vi "welcome.vi"   [LabVIEW 2018]
uses:
  user32.dll
types:
  T1 = enum32{"Invalid", "Standard", "Closed", "Hidden", "Minimized", "Maximized"}
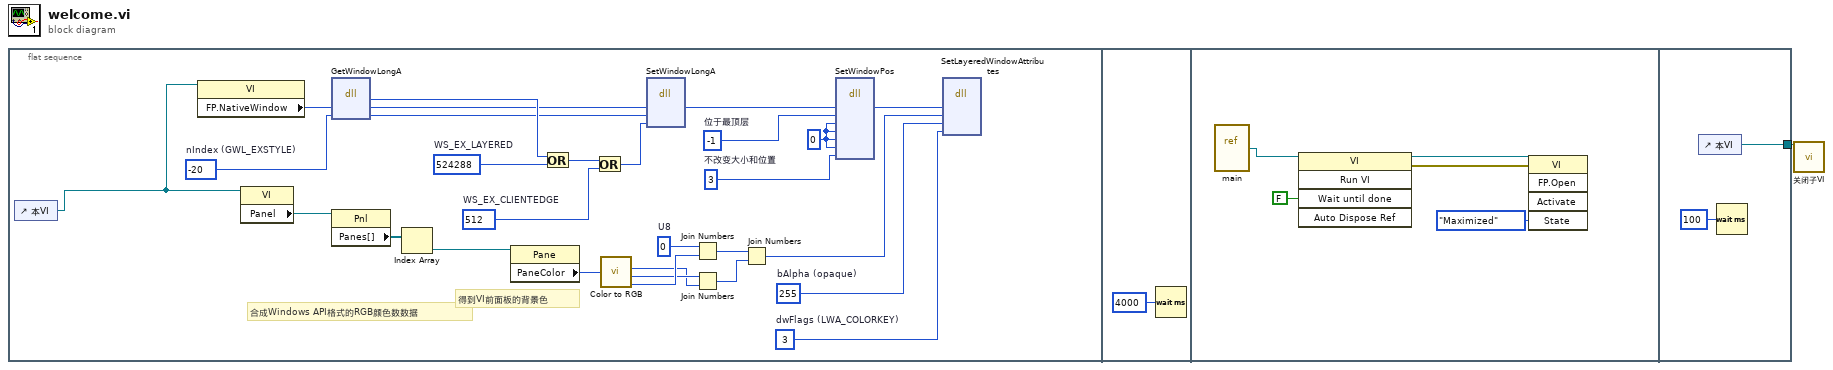
[diagram p0: block diagram]
diagram:
  n1 = flat-sequence {
    tunnel: [w36] -> w1
    frame #0 {
      w26 = 512  # WS_EX_CLIENTEDGE
      w22 = 3  # 不改变大小和位置
      w25 = 0 ("nIndex")
      w21 = -1  # 位于最顶层
      w3 = 255  # bAlpha (opaque)
      w2 = 3  # dwFlags (LWA_COLORKEY)
      w10 = u8 0  # U8
      w18 = 524288  # WS_EX_LAYERED
      w19 = -20  # nIndex (GWL_EXSTYLE)
      # "合成Windows API格式的RGB颜色数数据"
      # "得到VI前面板的背景色"
      n2 = control-ref of="本VI"() -> (w29:refnum<vi>)
      n3 = property class="VI"(reference=w29) -> ("FP.NativeWindow"=w20:u64)  [unwired: 1 in, 2 out]
      n4 = property class="VI"(reference=w29) -> ("Panel"=w5:refnum<vi>)  [unwired: 1 in, 2 out]
      n5 = dll-call lib="user32.dll" fn="GetWindowLongA"("handle"=w20, "nIndex"=w19) -> ("返回类型"=w17:i32, "handle"=w16:i32, "nIndex"=w15:i32)  [unwired: 3 in, 2 out]
      n6 = property class="Pnl"(reference=w5) -> ("Panes[]"=w6:refnum<vi>[])  [unwired: 1 in, 2 out]
      n7 = Index Array(array=w6) -> (element=w7:refnum<vi>)  [unwired: 1 in]
      n8 = property class="Pane"(reference=w7) -> ("PaneColor"=w11:u32)  [unwired: 1 in, 2 out]
      n9 = Or(x=w17, y=w18) -> (x .or. y?=w27:i32)
      n10 = Or(x=w27, y=w26) -> (x .or. y?=w28:i32)
      n11 = call <vilib>:"Color to RGB.vi"("Color"=w11) -> ("R"=w12:u8, "G"=w13:u8, "B"=w14:u8)  [unwired: 1 out]
      n12 = dll-call lib="USER32.DLL" fn="SetWindowLongA" label="SetWindowLong"("handle"=w16, "nIndex"=w15, "dwNewLong"=w28) -> ("handle"=w23:i32)  [unwired: 5 in, 3 out]
      n13 = Join Numbers(hi=w10, lo=w14) -> ((hi.lo)=w9:u16)
      n14 = Join Numbers(hi=w13, lo=w12) -> ((hi.lo)=w8:u16)
      n15 = Join Numbers(hi=w9, lo=w8) -> ((hi.lo)=w4:u32)
      n16 = dll-call lib="USER32.DLL" fn="SetWindowPos"("hWnd"=w23, "hWndInsertAfter"=w21, "x"=w25, "y"=w25, "cx"=w25, "cy"=w25, "wFlags"=w22) -> ("hWnd"=w24:i32)  [unwired: 9 in, 3 out]
      n17 = dll-call lib="USER32.DLL" fn="SetLayeredWindowAttributes" label="SetLayerdWindowAttributs"("handle"=w24, "crkey"=w4, "bAlpha"=w3, "dwFlags"=w2) -> ()  [unwired: 7 in, 3 out]
    }
    frame #1 {
      n18 = Wait (ms)(milliseconds to wait=u32 4000 ("等待时间（毫秒）")) -> ()  [unwired: 1 out]
    }
    frame #2 {
      n19 = vi-ref "main.vi"() -> (w31:refnum<vi>)
      n20 = invoke class="VI" method="Run VI"(reference=w31, "Wait until done"=FALSE ("结束前等待")) -> (reference out=w34:refnum<vi>, error out=w35:errorcluster)  [unwired: 3 in, 3 out]
      n21 = invoke class="VI" method="FP.Open"(reference=w34, error in=w35, "State"=T1."Maximized" ("状态")) -> ()  [unwired: 2 in, 5 out]
    }
    frame #3 {
      n22 = control-ref of="本VI"() -> (w36:refnum<vi>)
      n23 = Wait (ms)(milliseconds to wait=u32 100 ("等待时间（毫秒）")) -> ()  [unwired: 1 out]
    }
  }
  n24 = call "关闭子VI.vi"("引用"=w1) -> ()  [unwired: 9 in, 2 out]
